vi "Read file.vi"(11 "Text File in":refnum<class "Text File.lvclass">) -> (2 "file":refnum<file>, 3 "Text File out":refnum<class "Text File.lvclass">)   [LabVIEW 2019, in "TSC Event Logger.lvlib" / "Text File.lvclass"]
doc: "Data member access for the file reference.\n<b>Code Developed By:</b>\nTechnology Service Corporation\nBloomington, IN 47403\nwww.tsc.com/atcs\n\nDeveloper:\nDaniel Coons"
uses:
  Text File.lvclass
  Text File.lvclass/Text File.ctl
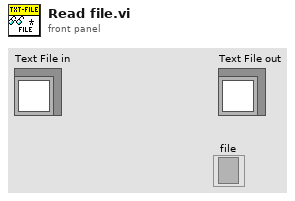
[diagram p1: front panel]
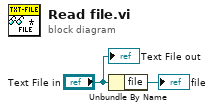
[diagram p0: block diagram]
diagram:
  n1 = Unbundle By Name("Text File in") -> ("file"=→"file":refnum<file>)
  "Text File out" <- "Text File in"
